vi "SetAcceleration.vi"(8 "error in":errorcluster, 9 "Acceleration":dbl, 10 "Axial #":i32, 11 "VISA resource":refnum<visa-resource-name>) -> (0 "error out":errorcluster)   [LabVIEW 2014, in "GRBLMotionCore.lvlib"]
uses:
  <instrlib>/GRBL/GRBLMotionCore.lvlib
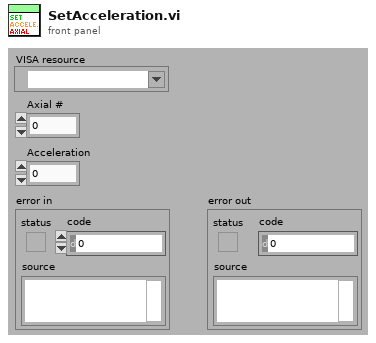
[diagram p1: front panel]
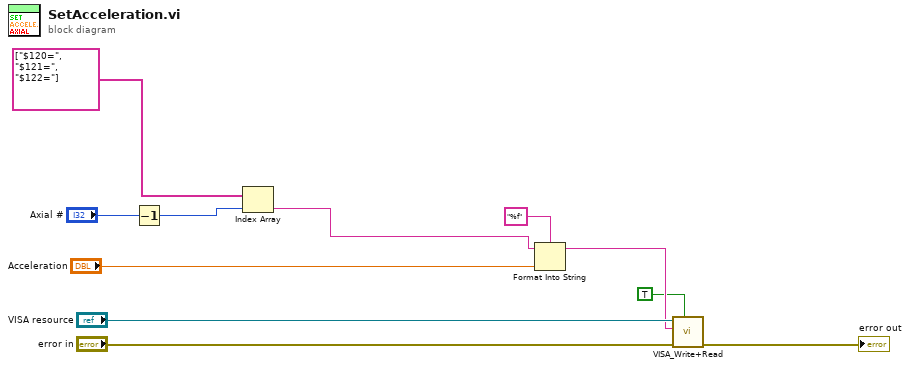
[diagram p0: block diagram]
diagram:
  n1 = Decrement(x="Axial #") -> (x-1=w4:i32)
  n2 = Index Array(array=string[] ["$120=", "$121=", "$122="], index=w4) -> (element=w1:string)
  n3 = Format Into String(format string="%f", initial string=w1, "Acceleration") -> (resulting string=w8:string)  [unwired: 1 in, 1 out]
  n4 = call <instrlib>:"VISA_Write+Read.vi"("Read? (T)"=TRUE ("Read?"), "error in (no error)"="error in", "Write Buffer"=w8, "VISA resource name"="VISA resource") -> ("error out"=→"error out":errorcluster)  [unwired: 5 in, 2 out]
